vi "DelWaveformALL.vi"() -> ()   [LabVIEW 2012]
panel:
  out "error out":errorcluster
  in  "串口参数设置":enum32{"常用设置", "不常用的"}(tab)
  in  "termination char\n(0xA = '\\n' = LF)":u8=10 caption="EOL字串-LF" format="%.0x"
  in  "flow control":u16(ring) caption="流量控制" items=["None"=0, "XON/XOFF"=1, "RTS/CTS"=2, "DTR/DSR"=4]
  in  "data bits":u16=8 caption="数据位" min=5 max=8 step=1
  in  "stop bits":u16(ring)=10 caption="停止位" items=["1.0"=10, "1.5"=15, "2.0"=20]
  in  "parity":u16(ring) caption="奇偶校验" items=["None", "Odd", "Even", "Mark", "Space"]
  in  "baud rate":u32=9600 caption="波特率"
  in  "VISA resource name":refnum<visa-resource-name>="COM1" caption="端口号"
  in  "timeout (ms)":u32=10000
  in  "XON Character":u8=17 format="%.0x"
  in  "XOFF Character":u8=19 format="%.0x"
  in  "Input buffer size":u32=4096 caption="输入缓冲区大小"
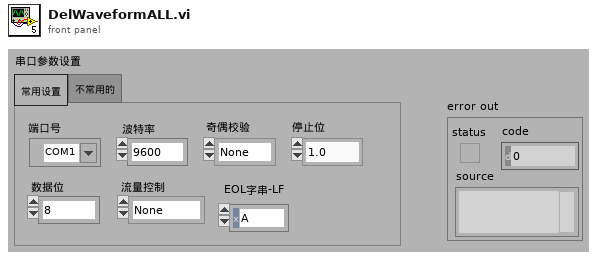
[diagram p1: front panel]
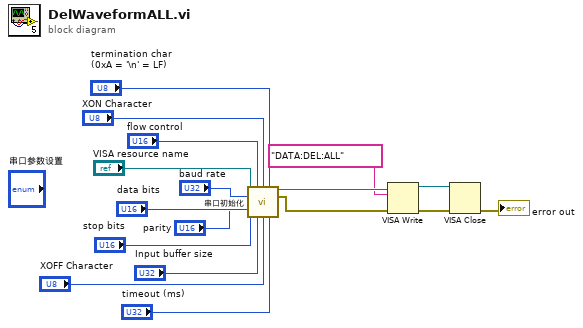
[diagram p0: block diagram]
diagram:
  n1 = call "串口初始化.vi"("VISA resource name"="VISA resource name", "flow control"="flow control", "XON Character"="XON Character", "termination char\n(0xA = '\\n' = LF)"="termination char\n(0xA = '\\n' = LF)", "baud rate"="baud rate", "data bits"="data bits", "parity"="parity", "stop bits"="stop bits", "Input buffer size"="Input buffer size", "XOFF Character"="XOFF Character", "timeout (ms)"="timeout (ms)") -> ("VISA resource name out"=w6:refnum<visa-resource-name>, "错误输出"=w5:errorcluster)  [unwired: 3 in]
  n2 = VISA Write(VISA resource name=w6, write buffer="DATA:DEL:ALL" ("写入缓冲区"), error in (no error)=w5) -> (VISA resource name out=w2:refnum<visa-resource-name>, error out=w3:errorcluster)  [unwired: 1 out]
  n3 = VISA Close(VISA resource name=w2, error in (no error)=w3) -> (error out=→"error out":errorcluster)
